vi "Get Notifiers.vi"(8 "error in (no error)":errorcluster, 10 "Reply Queue":refnum<queue>, 11 "PID Loop in":refnum<class "PID Loop.lvclass">) -> (0 "error out":errorcluster, 3 "PID Loop out":refnum<class "PID Loop.lvclass">)   [LabVIEW 2024, in "PID Loop.lvlib" / "PID Loop.lvclass"]
uses:
  PID Loop.lvclass
  PID Loop.lvclass/PID Loop.ctl
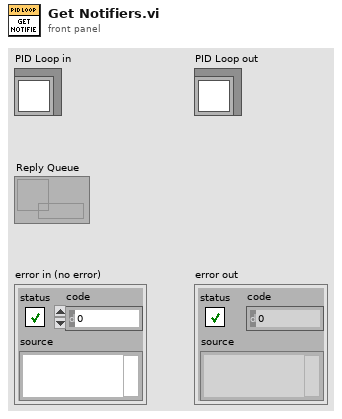
[diagram p1: front panel]
types:
  T1 = cluster{"Setpoint":refnum<notifier>, "Process Variable":refnum<notifier>, "Output":refnum<notifier>}
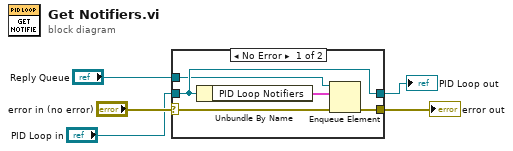
[diagram p0: block diagram]
diagram:
  n1 = case shown="No Error" "error in (no error)" {
    selector: "error in (no error)" -> [w7 w12]
    tunnel: [w6 w12] -> w4
    tunnel: [w10 w11] -> w2
    tunnel: "PID Loop in" -> [w10 w11]
    tunnel: "Reply Queue" -> [w9 _]
    frame No Error {
      n2 = Unbundle By Name(w10) -> ("PID Loop Notifiers"=w8:T1)
      n3 = Enqueue Element(queue=w9, element=w8, error in (no error)=w7) -> (error out=w6:errorcluster)  [unwired: 1 in, 2 out]
    }
    frame Error {
    }
  }
  "error out" <- w4
  "PID Loop out" <- w2
